vi "Read Tracker Msg.vi"(8 "error in (no error)":errorcluster, 11 "Data Tracker Msg in":refnum<class "Data Tracker Msg.lvclass">) -> (0 "error out":errorcluster, 1 "Timeout if Waiting":i32=-1, 2 "Send Function":T3=enum."Await Reply", 3 "Data Tracker Msg out":refnum<class "Data Tracker Msg.lvclass">, 4 "Message Priority":T2=enum."Normal", 5 "Publish Data?":bool=TRUE, 7 "Action":T1)   [LabVIEW 2020, in "Data Tracker.lvlib" / "Data Tracker Msg.lvclass"]
doc: "Read the private data of the Data Tracker Msg."
uses:
  Data Tracker Msg.lvclass
  PPL/HDH.Actor Framework.Core.Publisher.lvlibp/Messages/Response Msg/Response Core/Controls/Ctl_SendFunction.ctl
  PPL/HDH.Actor Framework.Core.Actor.lvlibp/1abvi3w/vi.lib/ActorFramework/Message Enqueuer/Message Priority.ctl
  Controls/Ctl_Action.ctl
  Data Tracker Msg.lvclass/Data Tracker Msg.ctl
  PPL/HDH.Actor Framework.Core.Publisher.lvlibp
  PPL/HDH.Actor Framework.Core.Actor.lvlibp/1abvi3w/vi.lib/ActorFramework/Message Enqueuer/Message Enqueuer.lvclass
  Data Tracker.lvlib
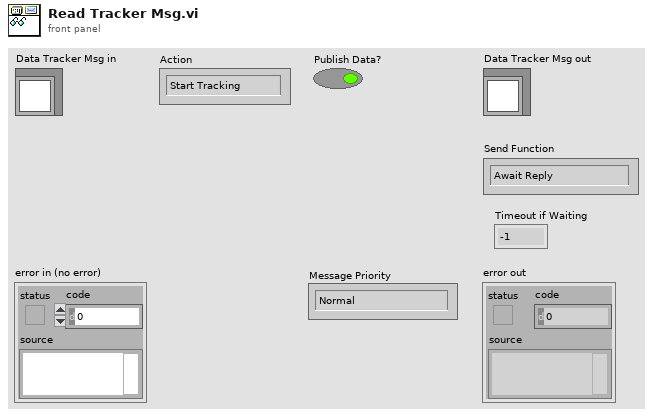
[diagram p1: front panel]
types:
  T1 = typedef "Data Tracker.lvlib/Ctl_Action.ctl" = enum16{"Start Tracking", "End Tracking", "Abort Tracking"}
  T2 = typedef "HDH.Actor Framework.Core.Actor.lvlibp/Message Enqueuer.lvclass/Message Priority.ctl" = enum16{"Low", "Normal", "High"}
  T3 = typedef "HDH.Actor Framework.Core.Publisher.lvlibp/Ctl_SendFunction.ctl" = enum16{"Send and Forget", "Request Reply", "Await Reply"}
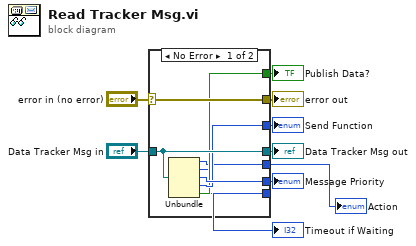
[diagram p0: block diagram]
diagram:
  n1 = case shown="No Error" "error in (no error)" {
    selector: "error in (no error)" -> [w16 w17]
    tunnel: [w16 w17] -> w8
    tunnel: [w15 w18] -> w6
    tunnel: "Data Tracker Msg in" -> [w15 w18]
    tunnel: [w13 _] -> w5
    tunnel: [w12 _] -> w4
    tunnel: [w11 _] -> w3
    tunnel: [w14 _] -> w2
    tunnel: [w10 _] -> w1
    frame No Error {
      n2 = Unbundle(w15) -> (w10:T1, w11:i32, w14:T2, w13:T3, w12:bool)
    }
    frame Error {
    }
  }
  "error out" <- w8
  "Data Tracker Msg out" <- w6
  "Send Function" <- w5
  "Timeout if Waiting" <- w3
  "Publish Data?" <- w4
  "Message Priority" <- w2
  "Action" <- w1
